vi "Array Point to RowCol.vi"(6 "Element Gap?":bool, 7 "Border Width":i32(ring)=3 items=["Classic"=3, "Modern"=4], 8 "error in":errorcluster, 9 "Mouse Coords":cluster{"Horizontal":i32, "Vertical":i32}, 11 "Array Ref":refnum<vi>) -> (0 "error out":errorcluster, 1 "Clicked Index":i32[](array[numeric]), 2 "Within Bounds?":bool, 3 "dup Ref":refnum<vi>)   [LabVIEW 2021]
doc: "Converts a pixel coordinate to an index into the array. Returns an array of indices with a length equal to the number of dimensions in the array. This method also returns whether the point is inside the bounds of the content rectangle.\n\nDownloaded from forum post to adapt to this application.\n\nWritten by J. David Saunders\nhttps://forums.ni.com/t5/LabVIEW/get-index-of-an-element-from-an-array-on-mouse-click/td-p/1310143/page/2"
panel:
  # "Written by J. David Saunders"
  # "https://forums.ni.com/t5/LabVIEW/get-index-of-an-element-from-an-array-on-mouse-click/td-p/1310143/page/2"
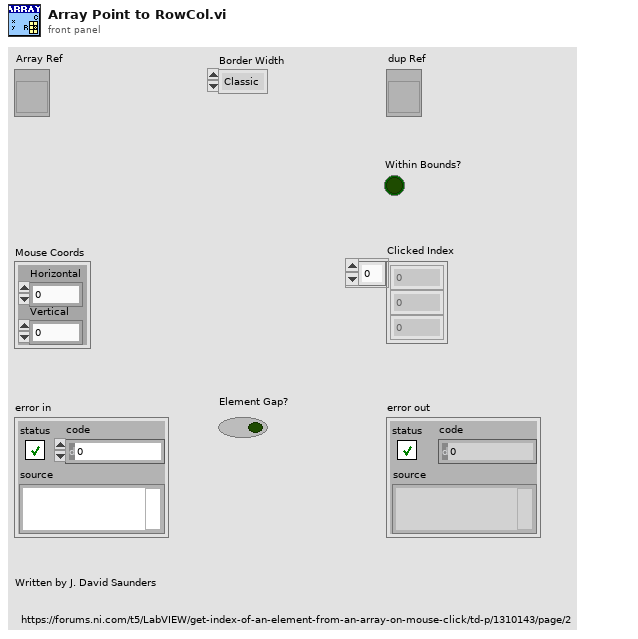
[diagram p1: front panel]
types:
  T1 = typedef "LVBoundsTypeDef.ctl" = cluster{"Width":u32, "Height":u32}
  T2 = cluster{"Number of Columns":u32, "Number of Rows":u32}
  T3 = cluster{"Number of Columns":i32, "Number of Rows":i32}
  T4 = typedef "LVPositionTypeDef.ctl" = cluster{"Left":i32, "Top":i32}
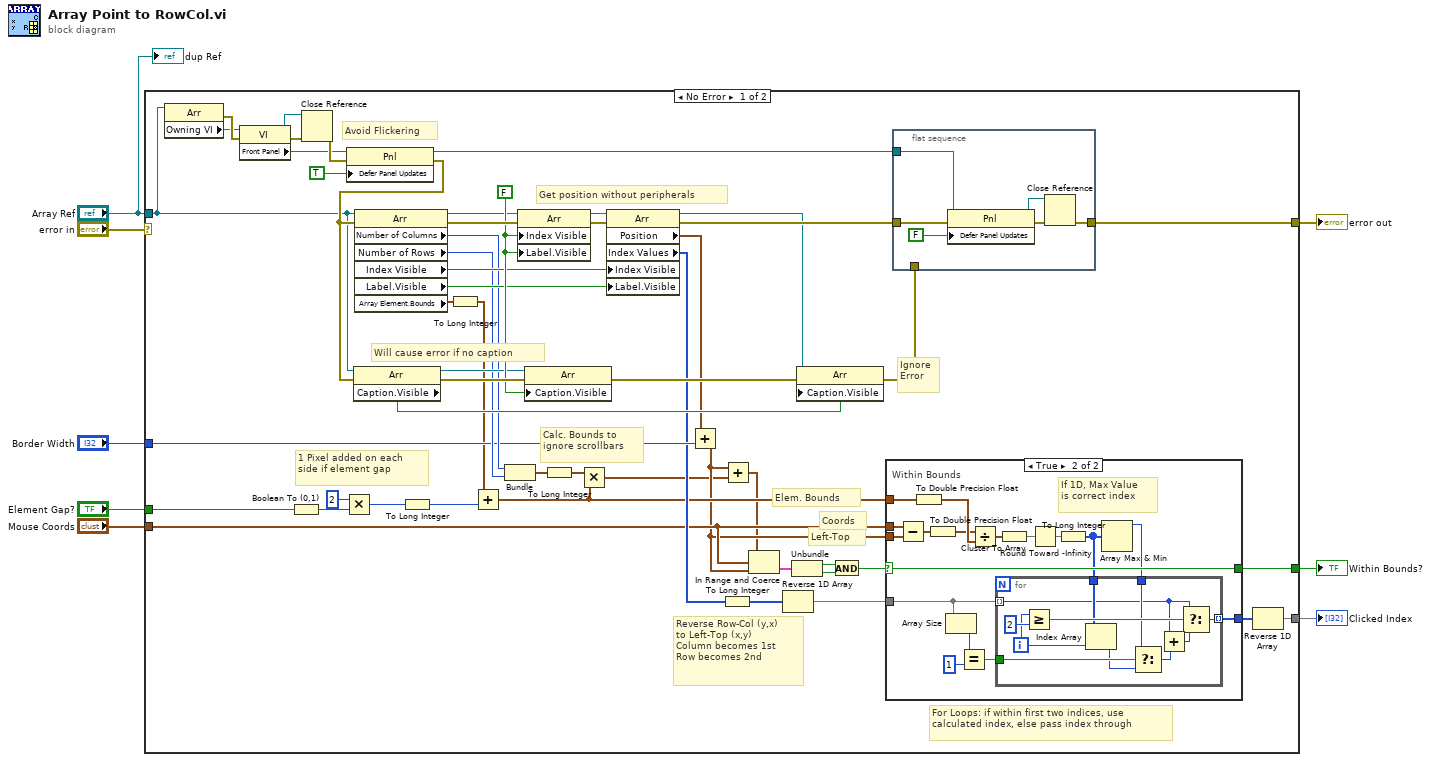
[diagram p0: block diagram]
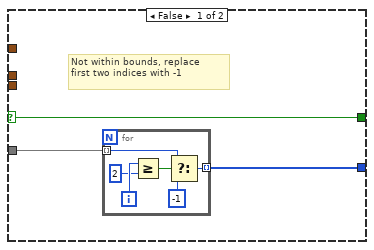
[diagram p2: hidden frame]
diagram:
  n1 = case shown="No Error" "error in" {
    selector: "error in" -> [_ w105]
    tunnel: "Element Gap?" -> [w50 _]
    tunnel: "Array Ref" -> [w15 _]
    tunnel: "Mouse Coords" -> [w24 _]
    tunnel: "Border Width" -> [w33 _]
    tunnel: [w28 _] -> w2
    tunnel: [w53 w105] -> w7
    tunnel: [w21 _] -> w1
    frame No Error {
      w47 = FALSE
      # "Avoid Flickering"
      # "Calc. Bounds to\nignore scrollbars"
      # "For Loops: if within first two indices, use\ncalculated index, else pass index through"
      # "Reverse Row-Col (y,x)\nto Left-Top (x,y)\nColumn becomes 1st\nRow becomes 2nd"
      # "Left-Top"
      # "Coords"
      # "Elem. Bounds"
      # "Ignore\nError"
      # "Get position without peripherals"
      # "1 Pixel added on each\nside if element gap"
      # "Will cause error if no caption"
      n2 = property class="Arr"(reference=w15) -> (error out=w57:errorcluster, "Owning VI"=w16:refnum<vi>)  [unwired: 1 in, 1 out]
      n3 = property class="VI"(reference=w16, error in=w57) -> (reference out=w9:refnum<vi>, error out=w52:errorcluster, "Front Panel"=w17:refnum<vi>)
      n4 = Boolean To (0,1)(Boolean=w50) -> (0, 1=w49:i16)
      n5 = Close Reference(reference=w9, error in (no error)=w52) -> (error out=w51:errorcluster)
      n6 = Multiply(x=i16 2 ("y"), y=w49) -> (x*y=w38:i16)
      n7 = property class="Pnl"(reference=w17, error in=w51, "Defer Panel Updates"=TRUE) -> (reference out=w13:refnum<vi>, error out=w56:errorcluster)
      n8 = property class="Arr"(reference=w15, error in=w56) -> (reference out=w42:refnum<vi>, error out=w61:errorcluster, "Caption.Visible"=w40:bool)
      n9 = property class="Arr"(reference=w15, error in=w56) -> (reference out=w44:refnum<vi>, error out=w60:errorcluster, "Number of Columns"=w37:u32, "Number of Rows"=w36:u32, "Index Visible"=w46:bool, "Label.Visible"=w45:bool, "Array Element.Bounds"=w39:T1)
      n10 = To Long Integer(number=w38) -> (32bit integer=w12:i32)
      n11 = To Long Integer(number=w39) -> (32bit integer=w11:cluster{"Width":i32, "Height":i32})
      n12 = Add(x=w11, y=w12) -> (x+y=w23:cluster{"Width":i32, "Height":i32})
      n13 = Bundle("Number of Columns"=w37, "Number of Rows"=w36) -> (w35:T2)  [unwired: 1 in]
      n14 = property class="Arr"(reference=w44, error in=w60, "Index Visible"=w47, "Label.Visible"=w47) -> (reference out=w43:refnum<vi>, error out=w59:errorcluster)
      n15 = property class="Arr"(reference=w42, error in=w61, "Caption.Visible"=w47) -> (error out=w58:errorcluster)  [unwired: 1 out]
      n16 = To Long Integer(number=w35) -> (32bit integer=w10:T3)
      n17 = Multiply(x=w10, y=w23) -> (x*y=w19:cluster{i32, i32})
      n18 = property class="Arr"(reference=w43, error in=w59, "Index Visible"=w46, "Label.Visible"=w45) -> (reference out=w41:refnum<vi>, error out=w55:errorcluster, "Position"=w34:T4, "Index Values"=w27:u32[])
      n19 = Add(x=w34, y=w33) -> (x+y=w20:T4)
      n20 = To Long Integer(number=w27) -> (32bit integer=w25:i32[])
      n21 = Add(x=w20, y=w19) -> (x+y=w18:T4)
      n22 = In Range and Coerce(upper limit=w18, x=w24, lower limit=w20) -> (In Range?=w32:cluster{"Left":bool, "Top":bool})  [unwired: 1 out]
      n23 = Reverse 1D Array(array=w25) -> (reversed array=w26:i32[])
      n24 = Unbundle(w32) -> ("Left"=w31:bool, "Top"=w30:bool)
      n25 = property class="Arr"(reference=w41, error in=w58, "Caption.Visible"=w40) -> (error out=w54:errorcluster)  [unwired: 1 out]
      n26 = And(x=w31, y=w30) -> (x .and. y?=w29:bool)
      n27 = case "Within Bounds" shown="True" w29 {
        selector: w29 -> [w70 w93]
        tunnel: [w70 w93] -> w28
        tunnel: w26 -> [w69 w84]
        tunnel: w24 -> [_ w92]
        tunnel: w23 -> [_ w89]
        tunnel: w20 -> [_ w91]
        tunnel: [w68 w87] -> w22
        frame False {
          # "Not within bounds, replace\nfirst two indices with -1"
          n28 = for {
            tunnel: w69 -> [w73] mode=indexing
            tunnel: [w71] -> w68 mode=indexing
            i -> [w76]
            n29 = Greater Or Equal?(x=w76, y=2) -> (x >= y?=w74:bool)
            n30 = Select(t=w73, s=w74, f=-1) -> (s? t:f=w71:i32)
          }
        }
        frame True {
          # "If 1D, Max Value\nis correct index"
          n31 = Subtract(x=w92, y=w91) -> (x-y=w90:T4)
          n32 = To Double Precision Float(number=w89) -> (double precision float=w78:cluster{"Width":dbl, "Height":dbl})
          n33 = To Double Precision Float(number=w90) -> (double precision float=w77:cluster{"Left":dbl, "Top":dbl})
          n34 = Array Size(array=w84) -> (size(s)=w83:i32)
          n35 = Equal?(x=w83, y=1) -> (x = y?=w81:bool)
          n36 = Divide(x=w77, y=w78) -> (x/y=w88:cluster{dbl, dbl})
          n37 = Cluster To Array(cluster=w88) -> (array=w80:dbl[])
          n38 = Round Toward -Infinity(1:w80) -> (0:w79:dbl[])
          n39 = To Long Integer(number=w79) -> (32bit integer=w86:i32[])
          n40 = Array Max & Min(array=w86) -> (max value=w85:i32)  [unwired: 3 out]
          n41 = for {
            tunnel: w84 -> [w95] mode=indexing
            tunnel: w86 -> [w101]
            tunnel: [w102] -> w87 mode=indexing
            tunnel: w85 -> [w98]
            tunnel: w81 -> [w99]
            i -> [w100]
            n42 = Greater Or Equal?(x=w100, y=2) -> (x >= y?=w103:bool)
            n43 = Index Array(array=w101, index=w100) -> (element=w97:i32)
            n44 = Select(t=w98, s=w99, f=w97) -> (s? t:f=w96:i32)
            n45 = Add(x=w95, y=w96) -> (x+y=w94:i32)
            n46 = Select(t=w95, s=w103, f=w94) -> (s? t:f=w102:i32)
          }
        }
      }
      n47 = flat-sequence {
        tunnel: w13 -> [w63]
        tunnel: w55 -> [w67]
        tunnel: w54 -> [_]
        tunnel: [w65] -> w53
        frame #0 {
          n48 = property class="Pnl"(reference=w63, error in=w67, "Defer Panel Updates"=FALSE) -> (reference out=w62:refnum<vi>, error out=w66:errorcluster)
          n49 = Close Reference(reference=w62, error in (no error)=w66) -> (error out=w65:errorcluster)
        }
      }
      n50 = Reverse 1D Array(array=w22) -> (reversed array=w21:i32[])
    }
    frame Error {
    }
  }
  "Clicked Index" <- w1
  "Within Bounds?" <- w2
  "error out" <- w7
  "dup Ref" <- "Array Ref"
